vi "Get Players Test App.vi"() -> ()   [LabVIEW 2013]
uses:
  LMH-Kodi.lvlib
  Player/Type Defs/Media Type.ctl
panel:
  out "Media Type":T1
  out "Error Out":errorcluster
  in  "Port (80)":u16=80
  in  "Hostname / IP":string="localhost"
  in  "Username":string="kodi"
  in  "Password":string
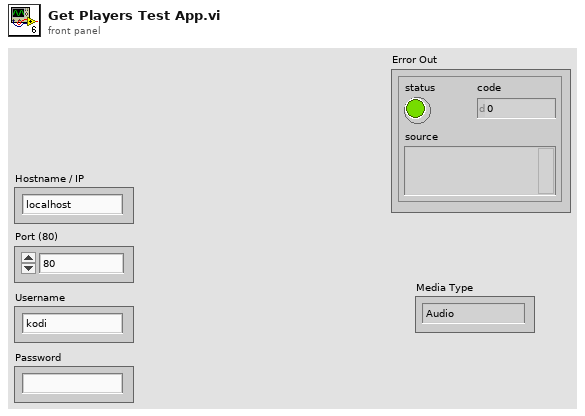
[diagram p1: front panel]
types:
  T1 = typedef "LMH-Kodi.lvlib/Player.lvlib/Media Type.ctl" = enum16{"Audio", "Video", "Picture", "None", "Error"}
  T2 = typedef "LMH-Kodi.lvlib/XBMC Ref.ctl" = cluster{"HTTP Handle":T3, "Hostname / IP":string, "jsonrpc":string}
  T3 = typedef "LabVIEWHTTPClient.lvlib/ClientHandle.ctl" = refnum<k1>
  T4 = typedef "LMH-Kodi.lvlib/Player.lvlib/Media Type.ctl" = enum8{"Audio", "Video", "Picture", "None", "Error"}
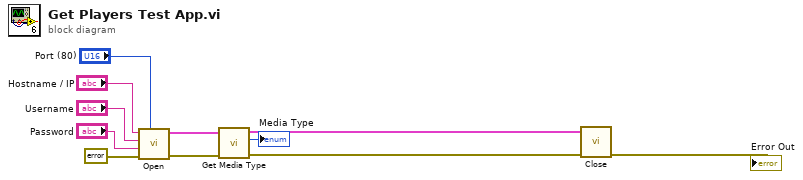
[diagram p0: block diagram]
diagram:
  n1 = call "Open.vi"("Port (80)"="Port (80)", "Error In"=errorcluster {"status"=FALSE, "code"=0, "source"=""}, "Password"="Password", "Username"="Username", "Hostname / IP"="Hostname / IP") -> ("Error Out"=w4:errorcluster, "XBMC Ref"=w5:T2)  [unwired: 5 in]
  n2 = call "Get Media Type.vi"("Error In"=w4, "XBMC Ref"=w5) -> ("Error Out"=w2:errorcluster, "Media Type"=→"Media Type":T4, "XBMC Ref"=w3:T2)  [unwired: 7 in]
  n3 = call "Close.vi"("Error In"=w2, "XBMC Ref"=w3) -> ("Error Out"=→"Error Out":errorcluster)  [unwired: 9 in]
